vi "rs3 Advanced set RSM control3.vi"(8 "error in (no error)":errorcluster, 10 "ST RSM":T1, 11 "device in":u64) -> (0 "error out":errorcluster, 1 "error":u64, 3 "Dev out":u64)   [LabVIEW 2017, in "libRealSense3.lvlib"]
doc: "This sets some register that affect the depth calculations"
uses:
  <vilib>/addons/RealSense/libRealSense3.lvlib
  Users/Greg McKaskle/Downloads/librealsense-1.12.1/librealsense-1.12.1/bin/Win32/realsense-d.dll
panel:
  # "RS3 Adv. Set RSM 2"
  # "(C) 2017 Intel Corp.,  AGJ"
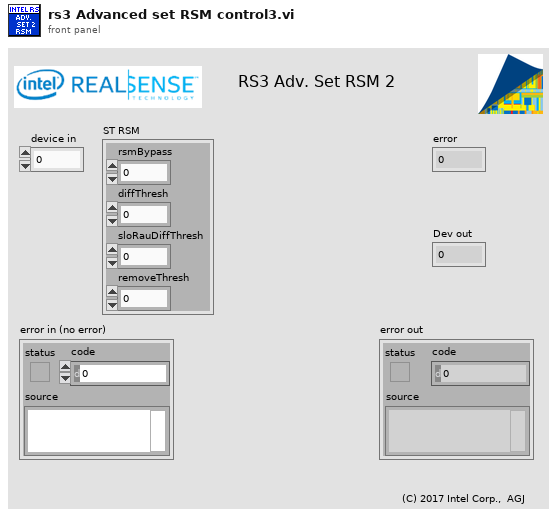
[diagram p1: front panel]
types:
  T1 = cluster{"rsmBypass":u32, "diffThresh":sgl, "sloRauDiffThresh":sgl, "removeThresh":u32}
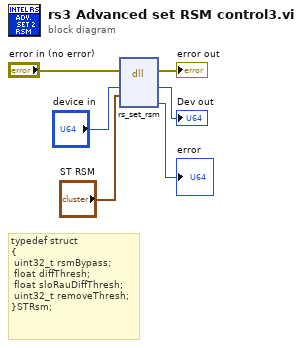
[diagram p0: block diagram]
diagram:
  # "typedef struct\n{\n\tuint32_t rsmBypass;\n\tfloat diffThresh;\n\tfloat sloRauDiffThresh;\n\tuint32_t removeThresh;\n}STRsm;"
  n1 = dll-call lib="C:/Users/Greg McKaskle/Downloads/librealsense-1.12.1/librealsense-1.12.1/bin/Win32/realsense-d.dll" fn="rs_set_rsm"(error in="error in (no error)", "device"="device in", "ST RSM"="ST RSM") -> (error out=→"error out":errorcluster, "device"=→"Dev out":u64, "error"=→"error":u64)  [unwired: 5 in, 1 out]
